vi "Get Instrument Type ID.vi"(8 "error in":errorcluster, 11 "session factory in":refnum<class "Session Factory.lvclass">) -> (0 "error out":errorcluster, 2 "instrument type id":string, 3 "session factory out":refnum<class "Session Factory.lvclass">)   [LabVIEW 2021, in "Session Management niDAQmx.lvlib" / "Session Factory.lvclass"]
doc: "Returns the type ID for the instrument in the pin map file. When using third party instruments not natively supported by the pin map editor, you must create a custom instrument in the pin map file and assign it a unique instrument type ID. Return the same instrument type ID from this method to access the third party instrument from within a measurement plug-in."
uses:
  Session Factory.lvclass
  Session Factory.lvclass/Session Factory.ctl
  Session Management niDAQmx.lvlib
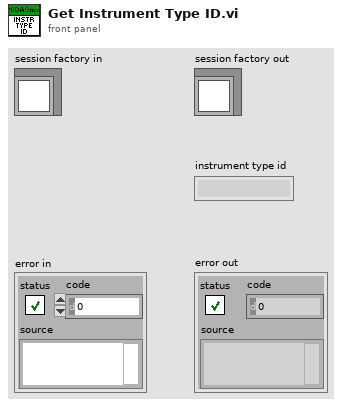
[diagram p1: front panel]
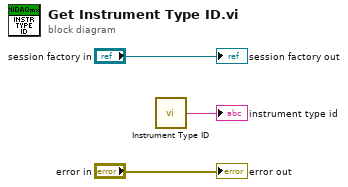
[diagram p0: block diagram]
diagram:
  n1 = call "Instrument Type ID.vi"() -> ("instrument type id"=→"instrument type id":string)  [unwired: 5 in]
  "error out" <- "error in"
  "session factory out" <- "session factory in"
